vi "MEMS_Controller.vi"(7 "ComCluster in":T7={"ComPort"="COM3", "ComPort_BaudRate"=115200, "ComPort_NDataBits"=8, "ComPort_Parity"=enum."None", "ComPort_NStopBits"=10} {"ComPort_NStopBits" items=["1.0"=10, "1.5"=15, "2.0"=20]; "ComPort_NDataBits" min=5 max=8 step=1}, 8 "error in (no error)":errorcluster, 9 "SignalInfo in":T3={"AScanPerBScan"=100.0, "BScanPerCScan"=100.0, "FastAxis"=enum."X-Axis", "SlowAxis"=enum."Y-Axis", "FastAxisFilter"=enum."NoFilter", "SlowAxisFilter"=enum."NoFilter", "AmpFastAxis"=1.0, "AmpSlowAxis"=1.0}, 10 "MCU_Config in":T6={"OctType"=enum."Spectrometer OCT", "ScanningMode"=enum."ContinuousScan", "AScanFrequency"=20000.0}, 11 "MEMS_Cmds":T8=enum."Run") -> (0 "error out":errorcluster={"status"=FALSE, "code"=1073676294, "source"="VISA Read in ComPort.vi->MEMS_Controller.vi"}, 1 "SignalInfo out":T3={"AScanPerBScan"=100.0, "BScanPerCScan"=100.0, "FastAxis"=enum."X-Axis", "SlowAxis"=enum."Y-Axis", "FastAxisFilter"=enum."NoFilter", "SlowAxisFilter"=enum."NoFilter", "AmpFastAxis"=1.0, "AmpSlowAxis"=1.0}, 2 "MCU_Config out":T6={"OctType"=enum."Spectrometer OCT", "ScanningMode"=enum."OneScan", "AScanFrequency"=20000.0}, 5 "ComCluster out":T7={"ComPort"="COM3", "ComPort_BaudRate"=115200, "ComPort_NDataBits"=8, "ComPort_Parity"=enum."None", "ComPort_NStopBits"=10})   [LabVIEW 2019]
uses:
  MEMS_CmdsTypeDef.ctl
  OCTTypeTypeDef.ctl
  ScanningModeTypeDef.ctl
  OutputStageTypeDef.ctl
  FilterTypeDef.ctl
  ComPortActionTypeDef.ctl
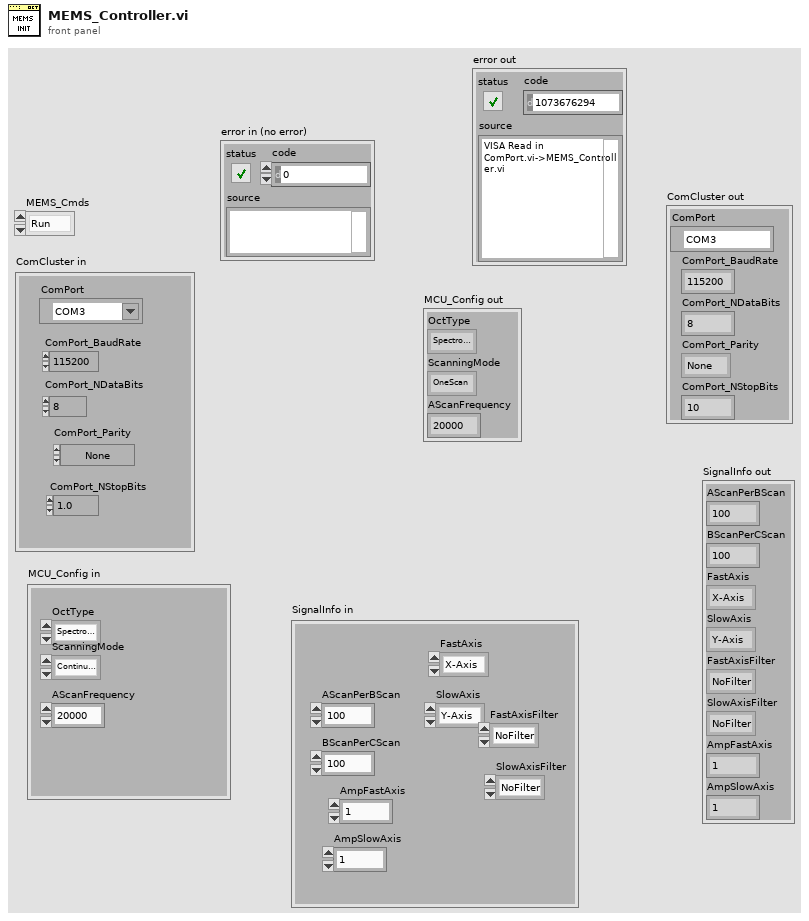
[diagram p1: front panel]
types:
  T1 = typedef "OutputStageTypeDef.ctl" = enum16{"X-Axis", "Y-Axis"}
  T2 = typedef "FilterTypeDef.ctl" = enum16{"IIR_Slow", "IIR_Fast", "NoFilter", "Bessel6thOrder300"}
  T3 = cluster{"AScanPerBScan":dbl, "BScanPerCScan":dbl, "FastAxis":T1, "SlowAxis":T1, "FastAxisFilter":T2, "SlowAxisFilter":T2, "AmpFastAxis":dbl, "AmpSlowAxis":dbl}
  T4 = typedef "OCTTypeTypeDef.ctl" = enum16{"Spectrometer OCT", "SSOCT"}
  T5 = typedef "ScanningModeTypeDef.ctl" = enum16{"OneScan", "ContinuousScan"}
  T6 = cluster{"OctType":T4, "ScanningMode":T5, "AScanFrequency":dbl}
  T7 = cluster{"ComPort":refnum<visa-resource-name>, "ComPort_BaudRate":u32, "ComPort_NDataBits":u16, "ComPort_Parity":enum16{"None", "Odd", "Even", "Mark", "Space"}, "ComPort_NStopBits":u16}
  T8 = typedef "MEMS_CmdsTypeDef.ctl" = enum16{"Init", "Config_AScan", "Config_BScan", "Config_CScan", "Run", "Stop", "Shutdown"}
  T9 = typedef "ComPortActionTypeDef.ctl" = enum16{"InitComPort", "ReadComPort", "WriteComePort", "CloseComPort"}
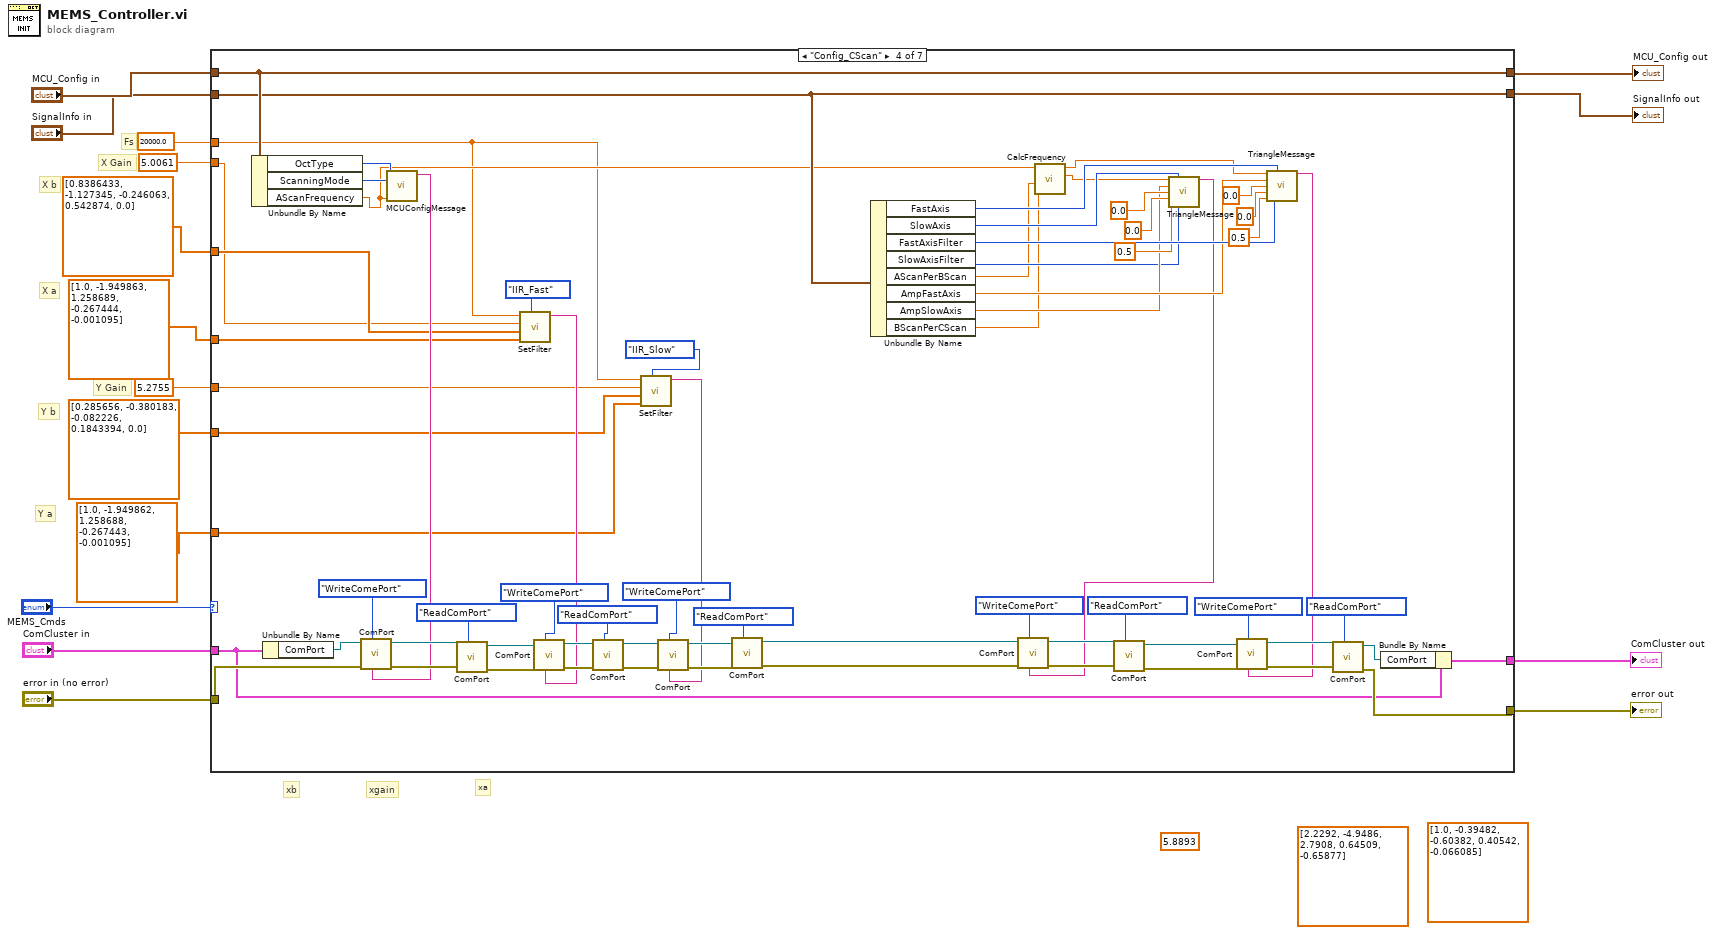
[diagram p0: block diagram]
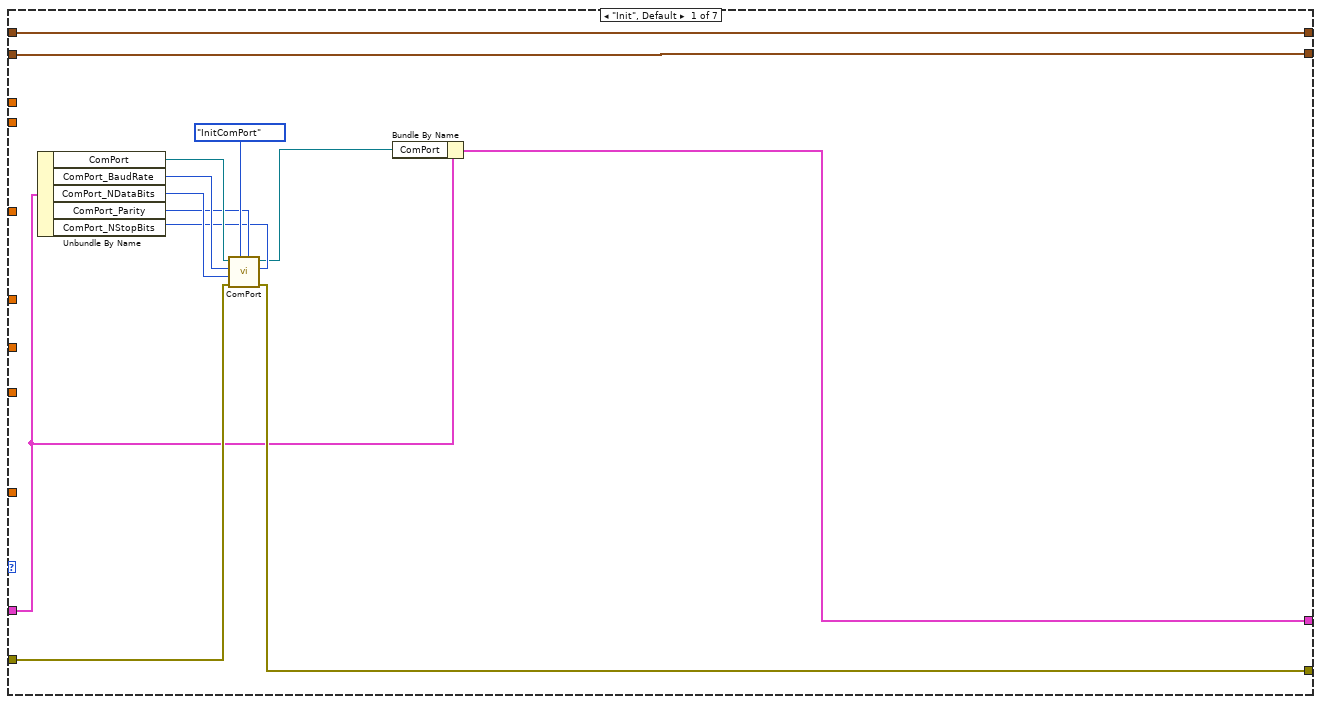
[diagram p2: hidden frame]
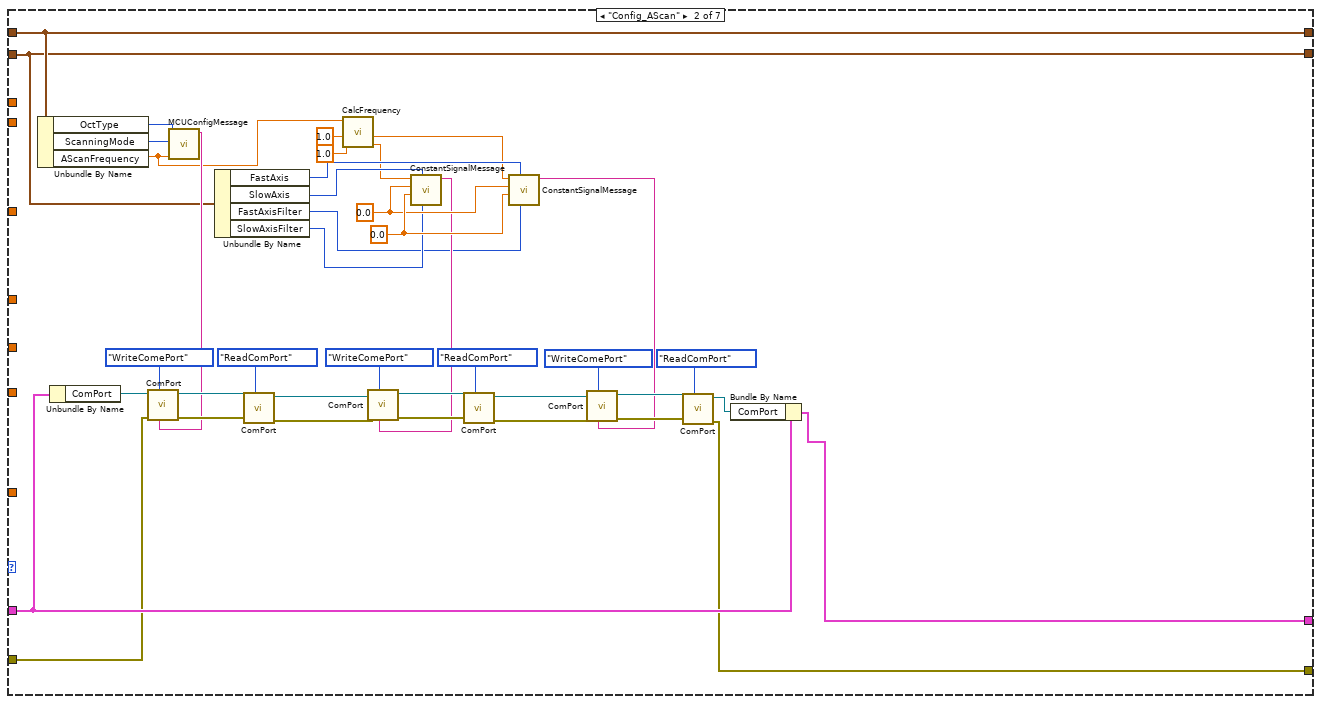
[diagram p3: hidden frame]
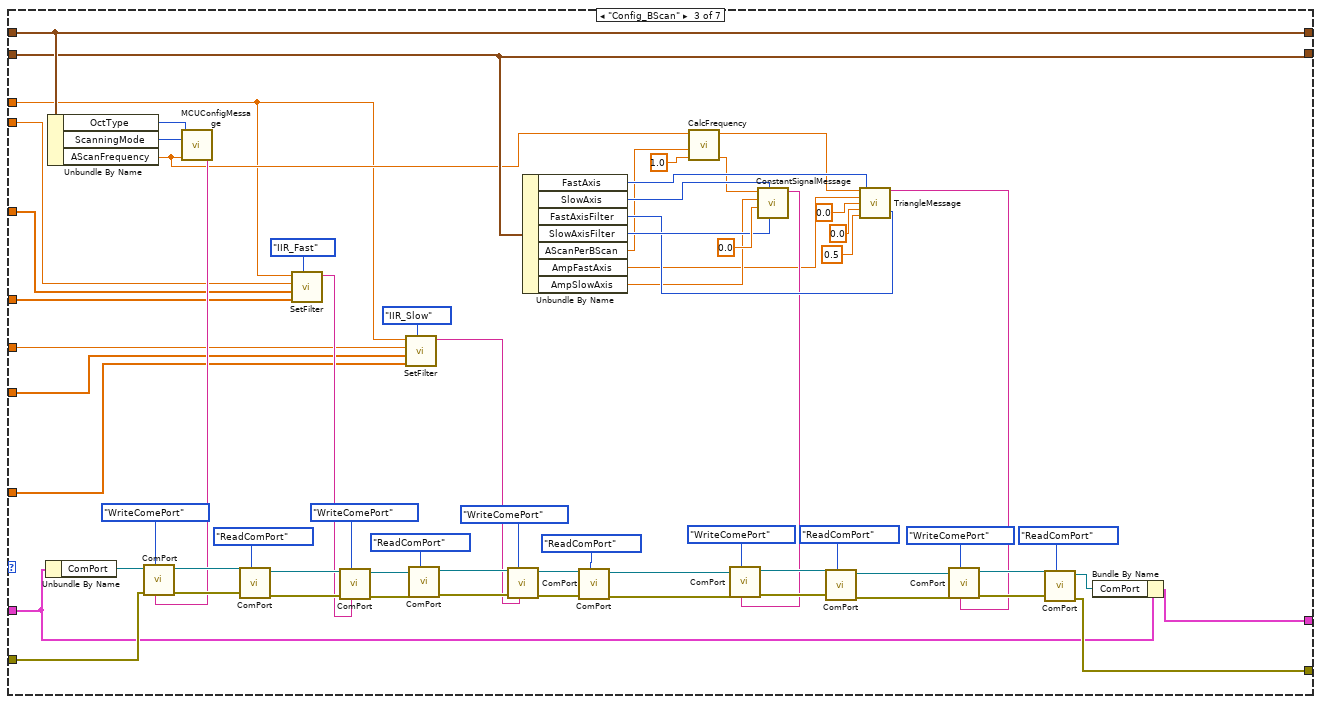
[diagram p4: hidden frame]
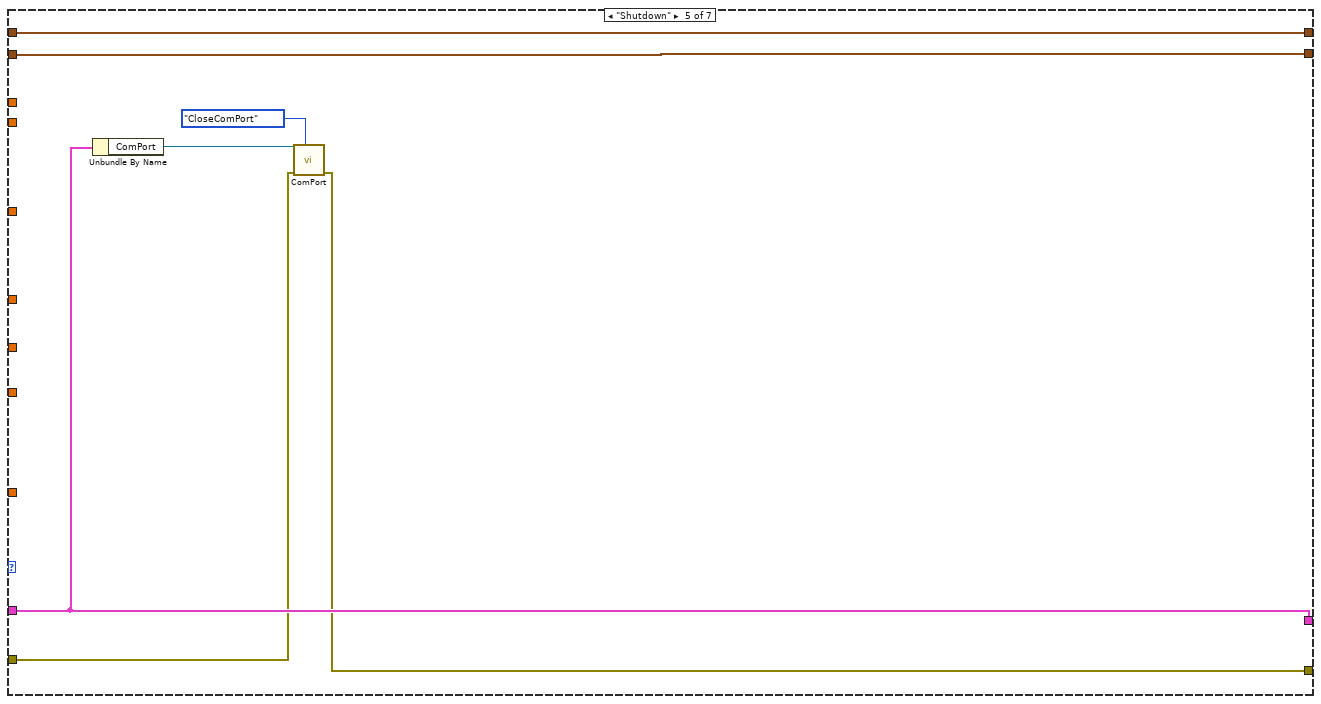
[diagram p5: hidden frame]
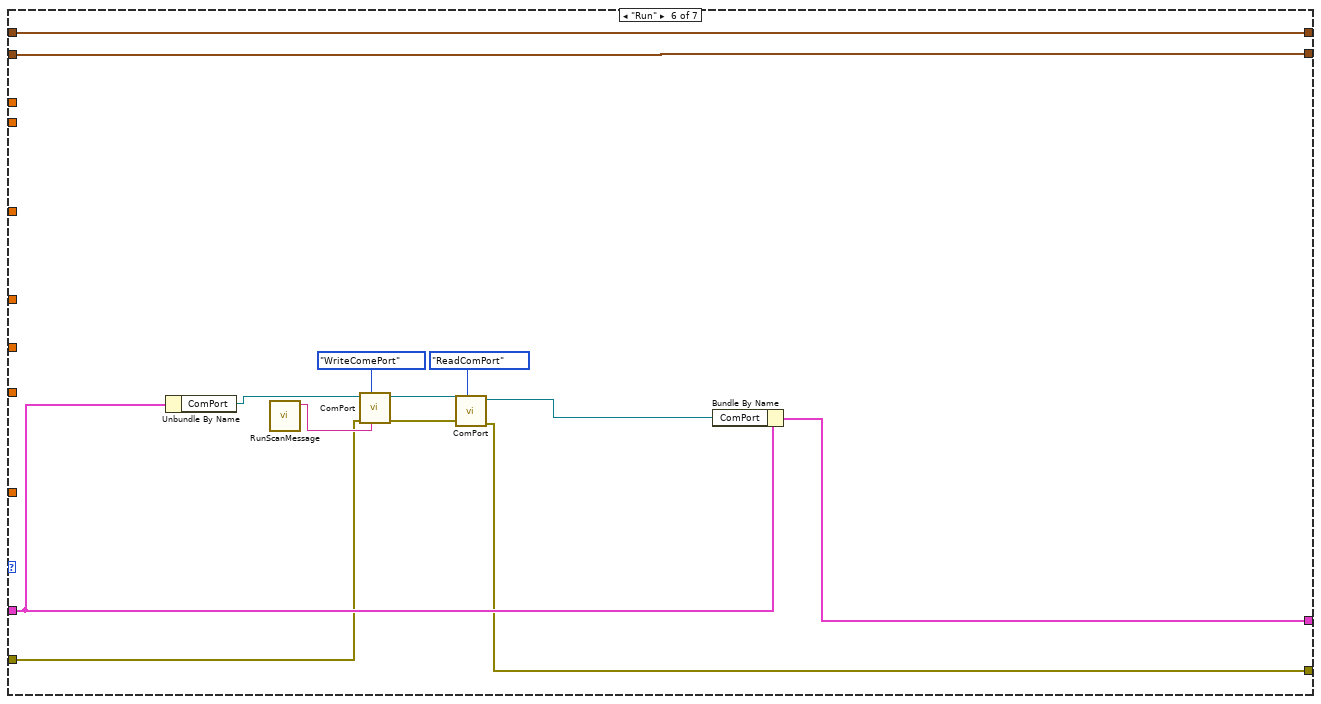
[diagram p6: hidden frame]
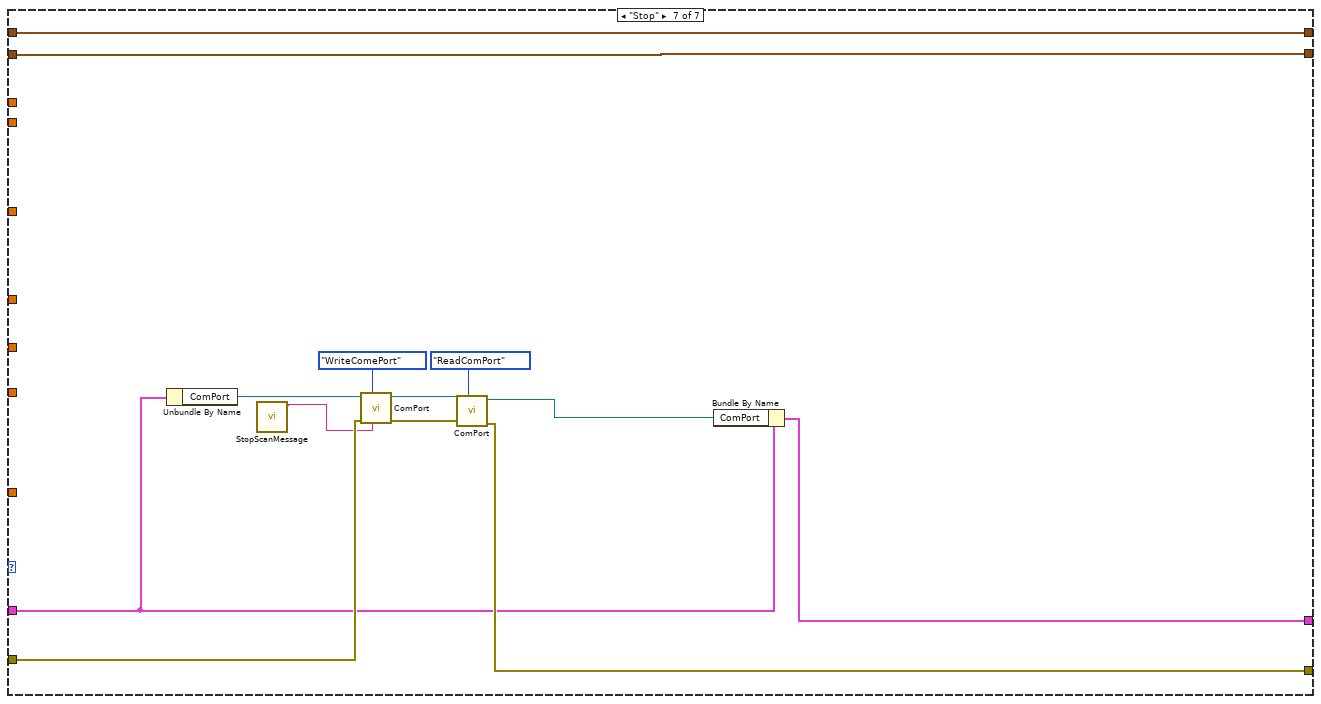
[diagram p7: hidden frame]
diagram:
  (unwired) dbl[] [1.0, -0.39482, -0.60382, 0.40542, -0.066085] ("a")
  (unwired) dbl[] [2.2292, -4.9486, 2.7908, 0.64509, -0.65877] ("b")
  (unwired) 5.8893 ("Gain")
  # "xgain"
  # "xa"
  # "xb"
  # "Y Gain"
  # "Fs"
  # "X Gain"
  # "Y a"
  # "Y b"
  # "X a"
  # "X b"
  n1 = case shown="\"Config_CScan\"" "MEMS_Cmds" {
    tunnel: "ComCluster in" -> [w20 w69 w117 w187 w212 w218 w229]
    tunnel: [w19 w68 w118 w186 w212 w219 w230] -> w12
    tunnel: "error in (no error)" -> [w23 w61 w120 w189 w210 w215 w232]
    tunnel: [w22 w55 w119 w188 w209 w214 w231] -> w13
    tunnel: "MCU_Config in" -> [w21 w36 w101 w168 w207 w225 w228]
    tunnel: [w21 w36 w101 w168 w207 w225 w228] -> w10
    tunnel: "SignalInfo in" -> [w17 w35 w100 w167 w206 w213 w226]
    tunnel: [w17 w35 w100 w167 w206 w213 w226] -> w8
    tunnel: dbl[] [1.0, -1.949863, 1.258689, -0.267444, -0.001095] ("a") -> [_ _ w74 w144 _ _ _]
    tunnel: dbl[] [0.8386433, -1.127345, -0.246063, 0.542874, 0.0] ("b") -> [_ _ w75 w143 _ _ _]
    tunnel: dbl[] [1.0, -1.949862, 1.258688, -0.267443, -0.001095] ("a") -> [_ _ w71 w142 _ _ _]
    tunnel: dbl[] [0.285656, -0.380183, -0.082226, 0.1843394, 0.0] ("b") -> [_ _ w72 w141 _ _ _]
    tunnel: 5.0061 ("Gain") -> [_ _ w76 w140 _ _ _]
    tunnel: 20000.0 ("SamplingFrequency") -> [_ _ w77 w139 _ _ _]
    tunnel: 5.2755 ("Gain") -> [_ _ w73 w138 _ _ _]
    frame "Init", Default {
      n2 = Unbundle By Name(w20) -> ("ComPort"=w28:refnum<visa-resource-name>, "ComPort_BaudRate"=w27:u32, "ComPort_NDataBits"=w26:u16, "ComPort_Parity"=w25:enum16{"None", "Odd", "Even", "Mark", "Space"}, "ComPort_NStopBits"=w24:u16)
      n3 = call "ComPort.vi"("stop bits (10: 1 bit)"=w24, "parity (0:none)"=w25, "ComAction"=ComPortActionTypeDef."InitComPort", "error in (no error)"=w23, "data bits (8)"=w26, "baud rate (9600)"=w27, "VISA resource name"=w28) -> ("error out"=w22:errorcluster, "VISA resource name out"=w18:refnum<visa-resource-name>)  [unwired: 2 in, 1 out]
      n4 = Bundle By Name(cluster=w20, "ComPort"=w18) -> (w19:T7)
    }
    frame "Config_AScan" {
      w44 = 0.0 ("Offset")
      w43 = 0.0 ("DC Value")
      n5 = Unbundle By Name(w36) -> ("OctType"=w47:T4, "ScanningMode"=w46:T5, "AScanFrequency"=w32:dbl)
      n6 = Unbundle By Name(w69) -> ("ComPort"=w54:refnum<visa-resource-name>)
      n7 = call "MCUConfigMessage.vi"("AScanFrequency"=w32, "ScanningMode"=w46, "OctType"=w47) -> ("MCUConfigMessage"=w45:string)  [unwired: 8 in]
      n8 = call "ComPort.vi"("write buffer"=w45, "ComAction"=ComPortActionTypeDef."WriteComePort", "error in (no error)"=w61, "VISA resource name"=w54) -> ("error out"=w60:errorcluster, "VISA resource name out"=w53:refnum<visa-resource-name>)  [unwired: 5 in, 1 out]
      n9 = Unbundle By Name(w35) -> ("FastAxis"=w40:T1, "SlowAxis"=w39:T1, "FastAxisFilter"=w37:T2, "SlowAxisFilter"=w38:T2)
      n10 = call "ComPort.vi"("ComAction"=ComPortActionTypeDef."ReadComPort", "error in (no error)"=w60, "VISA resource name"=w53) -> ("error out"=w59:errorcluster, "VISA resource name out"=w52:refnum<visa-resource-name>)  [unwired: 6 in, 1 out]
      n11 = call "CalcFrequency.vi"("BScanPerCScan"=1.0, "AScanPerBScan"=1.0, "AScanFrequency"=w32) -> ("SlowPeriod"=w33:dbl, "FastPeriod"=w34:dbl)  [unwired: 5 in, 2 out]
      n12 = call "ConstantSignalMessage.vi"("Filter"=w38, "OutputStage"=w39, "Offset"=w44, "DC Value"=w43, "Duration"=w33) -> ("ConstantSignalMessage"=w42:string)  [unwired: 6 in]
      n13 = call "ComPort.vi"("write buffer"=w42, "ComAction"=ComPortActionTypeDef."WriteComePort", "error in (no error)"=w59, "VISA resource name"=w52) -> ("error out"=w58:errorcluster, "VISA resource name out"=w51:refnum<visa-resource-name>)  [unwired: 5 in, 1 out]
      n14 = call "ComPort.vi"("ComAction"=ComPortActionTypeDef."ReadComPort", "error in (no error)"=w58, "VISA resource name"=w51) -> ("error out"=w57:errorcluster, "VISA resource name out"=w50:refnum<visa-resource-name>)  [unwired: 6 in, 1 out]
      n15 = call "ConstantSignalMessage.vi"("Filter"=w37, "OutputStage"=w40, "Offset"=w44, "DC Value"=w43, "Duration"=w34) -> ("ConstantSignalMessage"=w41:string)  [unwired: 6 in]
      n16 = call "ComPort.vi"("write buffer"=w41, "ComAction"=ComPortActionTypeDef."WriteComePort", "error in (no error)"=w57, "VISA resource name"=w50) -> ("error out"=w56:errorcluster, "VISA resource name out"=w49:refnum<visa-resource-name>)  [unwired: 5 in, 1 out]
      n17 = call "ComPort.vi"("ComAction"=ComPortActionTypeDef."ReadComPort", "error in (no error)"=w56, "VISA resource name"=w49) -> ("error out"=w55:errorcluster, "VISA resource name out"=w48:refnum<visa-resource-name>)  [unwired: 6 in, 1 out]
      n18 = Bundle By Name(cluster=w69, "ComPort"=w48) -> (w68:T7)
    }
    frame "Config_BScan" {
      n19 = Unbundle By Name(w117) -> ("ComPort"=w126:refnum<visa-resource-name>)
      n20 = Unbundle By Name(w101) -> ("OctType"=w116:T4, "ScanningMode"=w115:T5, "AScanFrequency"=w99:dbl)
      n21 = call "MCUConfigMessage.vi"("AScanFrequency"=w99, "ScanningMode"=w115, "OctType"=w116) -> ("MCUConfigMessage"=w111:string)  [unwired: 8 in]
      n22 = call "ComPort.vi"("write buffer"=w111, "ComAction"=ComPortActionTypeDef."WriteComePort", "error in (no error)"=w120, "VISA resource name"=w126) -> ("error out"=w130:errorcluster, "VISA resource name out"=w125:refnum<visa-resource-name>)  [unwired: 5 in, 1 out]
      n23 = call "ComPort.vi"("ComAction"=ComPortActionTypeDef."ReadComPort", "error in (no error)"=w130, "VISA resource name"=w125) -> ("error out"=w84:errorcluster, "VISA resource name out"=w89:refnum<visa-resource-name>)  [unwired: 6 in, 1 out]
      n24 = call "SetFilter.vi"("Filter"=FilterTypeDef."IIR_Fast", "a"=w74, "b"=w75, "Gain"=w76, "SamplingFrequency"=w77) -> ("SetFilterMessage"=w79:string)  [unwired: 6 in]
      n25 = call "ComPort.vi"("write buffer"=w79, "ComAction"=ComPortActionTypeDef."WriteComePort", "error in (no error)"=w84, "VISA resource name"=w89) -> ("error out"=w83:errorcluster, "VISA resource name out"=w88:refnum<visa-resource-name>)  [unwired: 5 in, 1 out]
      n26 = call "SetFilter.vi"("Filter"=FilterTypeDef."IIR_Slow", "a"=w71, "b"=w72, "Gain"=w73, "SamplingFrequency"=w77) -> ("SetFilterMessage"=w78:string)  [unwired: 6 in]
      n27 = call "ComPort.vi"("ComAction"=ComPortActionTypeDef."ReadComPort", "error in (no error)"=w83, "VISA resource name"=w88) -> ("error out"=w82:errorcluster, "VISA resource name out"=w87:refnum<visa-resource-name>)  [unwired: 6 in, 1 out]
      n28 = call "ComPort.vi"("write buffer"=w78, "ComAction"=ComPortActionTypeDef."WriteComePort", "error in (no error)"=w82, "VISA resource name"=w87) -> ("error out"=w81:errorcluster, "VISA resource name out"=w86:refnum<visa-resource-name>)  [unwired: 5 in, 1 out]
      n29 = Unbundle By Name(w100) -> ("FastAxis"=w110:T1, "SlowAxis"=w113:T1, "FastAxisFilter"=w109:T2, "SlowAxisFilter"=w112:T2, "AScanPerBScan"=w98:dbl, "AmpFastAxis"=w106:dbl, "AmpSlowAxis"=w107:dbl)
      n30 = call "ComPort.vi"("ComAction"=ComPortActionTypeDef."ReadComPort", "error in (no error)"=w81, "VISA resource name"=w86) -> ("error out"=w80:errorcluster, "VISA resource name out"=w85:refnum<visa-resource-name>)  [unwired: 6 in, 1 out]
      n31 = call "CalcFrequency.vi"("BScanPerCScan"=1.0, "AScanPerBScan"=w98, "AScanFrequency"=w99) -> ("SlowPeriod"=w96:dbl, "FastFrequency"=w95:dbl)  [unwired: 5 in, 2 out]
      n32 = call "ConstantSignalMessage.vi"("Filter"=w112, "OutputStage"=w113, "Offset"=0.0, "DC Value"=w107, "Duration"=w96) -> ("ConstantSignalMessage"=w108:string)  [unwired: 6 in]
      n33 = call "ComPort.vi"("write buffer"=w108, "ComAction"=ComPortActionTypeDef."WriteComePort", "error in (no error)"=w80, "VISA resource name"=w85) -> ("error out"=w129:errorcluster, "VISA resource name out"=w124:refnum<visa-resource-name>)  [unwired: 5 in, 1 out]
      n34 = call "ComPort.vi"("ComAction"=ComPortActionTypeDef."ReadComPort", "error in (no error)"=w129, "VISA resource name"=w124) -> ("error out"=w128:errorcluster, "VISA resource name out"=w123:refnum<visa-resource-name>)  [unwired: 6 in, 1 out]
      n35 = call "TriangleMessage.vi"("Frequency"=w95, "OutputStage"=w110, "Amplitude"=w106, "Phase"=0.0, "Offset"=0.0, "Width"=0.5, "Filter"=w109) -> ("TriangleSignalMessage"=w102:string)  [unwired: 8 in]
      n36 = call "ComPort.vi"("write buffer"=w102, "ComAction"=ComPortActionTypeDef."WriteComePort", "error in (no error)"=w128, "VISA resource name"=w123) -> ("error out"=w127:errorcluster, "VISA resource name out"=w122:refnum<visa-resource-name>)  [unwired: 5 in, 1 out]
      n37 = call "ComPort.vi"("ComAction"=ComPortActionTypeDef."ReadComPort", "error in (no error)"=w127, "VISA resource name"=w122) -> ("error out"=w119:errorcluster, "VISA resource name out"=w121:refnum<visa-resource-name>)  [unwired: 6 in, 1 out]
      n38 = Bundle By Name(cluster=w117, "ComPort"=w121) -> (w118:T7)
    }
    frame "Config_CScan" {
      n39 = Unbundle By Name(w168) -> ("OctType"=w185:T4, "ScanningMode"=w184:T5, "AScanFrequency"=w166:dbl)
      n40 = Unbundle By Name(w187) -> ("ComPort"=w195:refnum<visa-resource-name>)
      n41 = call "MCUConfigMessage.vi"("AScanFrequency"=w166, "ScanningMode"=w184, "OctType"=w185) -> ("MCUConfigMessage"=w172:string)  [unwired: 8 in]
      n42 = call "ComPort.vi"("write buffer"=w172, "ComAction"=ComPortActionTypeDef."WriteComePort", "error in (no error)"=w189, "VISA resource name"=w195) -> ("error out"=w199:errorcluster, "VISA resource name out"=w194:refnum<visa-resource-name>)  [unwired: 5 in, 1 out]
      n43 = call "ComPort.vi"("ComAction"=ComPortActionTypeDef."ReadComPort", "error in (no error)"=w199, "VISA resource name"=w194) -> ("error out"=w160:errorcluster, "VISA resource name out"=w161:refnum<visa-resource-name>)  [unwired: 6 in, 1 out]
      n44 = call "SetFilter.vi"("Filter"=FilterTypeDef."IIR_Fast", "a"=w144, "b"=w143, "Gain"=w140, "SamplingFrequency"=w139) -> ("SetFilterMessage"=w146:string)  [unwired: 6 in]
      n45 = call "ComPort.vi"("write buffer"=w146, "ComAction"=ComPortActionTypeDef."WriteComePort", "error in (no error)"=w160, "VISA resource name"=w161) -> ("error out"=w158:errorcluster, "VISA resource name out"=w159:refnum<visa-resource-name>)  [unwired: 5 in, 1 out]
      n46 = call "ComPort.vi"("ComAction"=ComPortActionTypeDef."ReadComPort", "error in (no error)"=w158, "VISA resource name"=w159) -> ("error out"=w156:errorcluster, "VISA resource name out"=w157:refnum<visa-resource-name>)  [unwired: 6 in, 1 out]
      n47 = call "SetFilter.vi"("Filter"=FilterTypeDef."IIR_Slow", "a"=w142, "b"=w141, "Gain"=w138, "SamplingFrequency"=w139) -> ("SetFilterMessage"=w145:string)  [unwired: 6 in]
      n48 = call "ComPort.vi"("write buffer"=w145, "ComAction"=ComPortActionTypeDef."WriteComePort", "error in (no error)"=w156, "VISA resource name"=w157) -> ("error out"=w154:errorcluster, "VISA resource name out"=w155:refnum<visa-resource-name>)  [unwired: 5 in, 1 out]
      n49 = call "ComPort.vi"("ComAction"=ComPortActionTypeDef."ReadComPort", "error in (no error)"=w154, "VISA resource name"=w155) -> ("error out"=w152:errorcluster, "VISA resource name out"=w153:refnum<visa-resource-name>)  [unwired: 6 in, 1 out]
      n50 = Unbundle By Name(w167) -> ("FastAxis"=w183:T1, "SlowAxis"=w170:T1, "FastAxisFilter"=w182:T2, "SlowAxisFilter"=w169:T2, "AScanPerBScan"=w165:dbl, "AmpFastAxis"=w181:dbl, "AmpSlowAxis"=w174:dbl, "BScanPerCScan"=w164:dbl)
      n51 = call "CalcFrequency.vi"("BScanPerCScan"=w164, "AScanPerBScan"=w165, "AScanFrequency"=w166) -> ("SlowFrequency"=w162:dbl, "FastFrequency"=w163:dbl)  [unwired: 5 in, 2 out]
      n52 = call "TriangleMessage.vi"("Frequency"=w162, "OutputStage"=w170, "Amplitude"=w174, "Phase"=0.0, "Offset"=0.0, "Width"=0.5, "Filter"=w169) -> ("TriangleSignalMessage"=w173:string)  [unwired: 8 in]
      n53 = call "ComPort.vi"("write buffer"=w173, "ComAction"=ComPortActionTypeDef."WriteComePort", "error in (no error)"=w152, "VISA resource name"=w153) -> ("error out"=w198:errorcluster, "VISA resource name out"=w193:refnum<visa-resource-name>)  [unwired: 5 in, 1 out]
      n54 = call "ComPort.vi"("ComAction"=ComPortActionTypeDef."ReadComPort", "error in (no error)"=w198, "VISA resource name"=w193) -> ("error out"=w197:errorcluster, "VISA resource name out"=w192:refnum<visa-resource-name>)  [unwired: 6 in, 1 out]
      n55 = call "TriangleMessage.vi"("Frequency"=w163, "OutputStage"=w183, "Amplitude"=w181, "Phase"=0.0, "Offset"=0.0, "Width"=0.5, "Filter"=w182) -> ("TriangleSignalMessage"=w171:string)  [unwired: 8 in]
      n56 = call "ComPort.vi"("write buffer"=w171, "ComAction"=ComPortActionTypeDef."WriteComePort", "error in (no error)"=w197, "VISA resource name"=w192) -> ("error out"=w196:errorcluster, "VISA resource name out"=w191:refnum<visa-resource-name>)  [unwired: 5 in, 1 out]
      n57 = call "ComPort.vi"("ComAction"=ComPortActionTypeDef."ReadComPort", "error in (no error)"=w196, "VISA resource name"=w191) -> ("error out"=w188:errorcluster, "VISA resource name out"=w190:refnum<visa-resource-name>)  [unwired: 6 in, 1 out]
      n58 = Bundle By Name(cluster=w187, "ComPort"=w190) -> (w186:T7)
    }
    frame "Shutdown" {
      n59 = Unbundle By Name(w212) -> ("ComPort"=w211:refnum<visa-resource-name>)
      n60 = call "ComPort.vi"("ComAction"=ComPortActionTypeDef."CloseComPort", "error in (no error)"=w210, "VISA resource name"=w211) -> ("error out"=w209:errorcluster)  [unwired: 6 in, 2 out]
    }
    frame "Run" {
      n61 = Unbundle By Name(w218) -> ("ComPort"=w220:refnum<visa-resource-name>)
      n62 = call "RunScanMessage.vi"() -> ("RunScanMessage"=w216:string)  [unwired: 11 in]
      n63 = call "ComPort.vi"("write buffer"=w216, "ComAction"=ComPortActionTypeDef."WriteComePort", "error in (no error)"=w215, "VISA resource name"=w220) -> ("error out"=w222:errorcluster, "VISA resource name out"=w221:refnum<visa-resource-name>)  [unwired: 5 in, 1 out]
      n64 = call "ComPort.vi"("ComAction"=ComPortActionTypeDef."ReadComPort", "error in (no error)"=w222, "VISA resource name"=w221) -> ("error out"=w214:errorcluster, "VISA resource name out"=w217:refnum<visa-resource-name>)  [unwired: 6 in, 1 out]
      n65 = Bundle By Name(cluster=w218, "ComPort"=w217) -> (w219:T7)
    }
    frame "Stop" {
      n66 = Unbundle By Name(w229) -> ("ComPort"=w234:refnum<visa-resource-name>)
      n67 = call "StopScanMessage.vi"() -> ("StopScanMessage"=w227:string)  [unwired: 11 in]
      n68 = call "ComPort.vi"("write buffer"=w227, "ComAction"=ComPortActionTypeDef."WriteComePort", "error in (no error)"=w232, "VISA resource name"=w234) -> ("error out"=w236:errorcluster, "VISA resource name out"=w235:refnum<visa-resource-name>)  [unwired: 5 in, 1 out]
      n69 = call "ComPort.vi"("ComAction"=ComPortActionTypeDef."ReadComPort", "error in (no error)"=w236, "VISA resource name"=w235) -> ("error out"=w231:errorcluster, "VISA resource name out"=w233:refnum<visa-resource-name>)  [unwired: 6 in, 1 out]
      n70 = Bundle By Name(cluster=w229, "ComPort"=w233) -> (w230:T7)
    }
  }
  "error out" <- w13
  "ComCluster out" <- w12
  "MCU_Config out" <- w10
  "SignalInfo out" <- w8
